vi "Fehler Auswerten.vi"(9 "Max Fehler in %":dbl, 10 "setpoint":dbl, 11 "output":dbl) -> (3 "Error":bool)   [LabVIEW 2020, in "Linearisierung v2.lvlib" / "Gasteiler.lvlib" / "HovaCAL_Interface.lvlib"]
uses:
  HovaCAL_Interface.lvlib
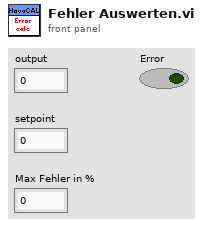
[diagram p1: front panel]
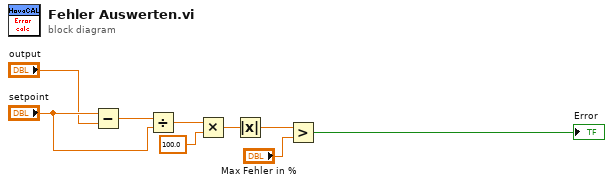
[diagram p0: block diagram]
diagram:
  n1 = Subtract(x="setpoint", y="output") -> (x-y=w2:dbl)
  n2 = Divide(x=w2, y="setpoint") -> (x/y=w4:dbl)
  n3 = Multiply(x=w4, y=100.0) -> (x*y=w6:dbl)
  n4 = Absolute Value(x=w6) -> (abs(x)=w7:dbl)
  n5 = Greater?(x=w7, y="Max Fehler in %") -> (0:→"Error":bool)
